vi "Single Shot Camera Test.vi"() -> ()   [LabVIEW 2017]
uses:
  IMAQCV/IMAQCV.lvlib
  IMAQCV/LVOpenCV.lvlib
panel:
  in  "Image Size":T1(ring)
  out "Gray picture":picture
  out "Color picture":picture
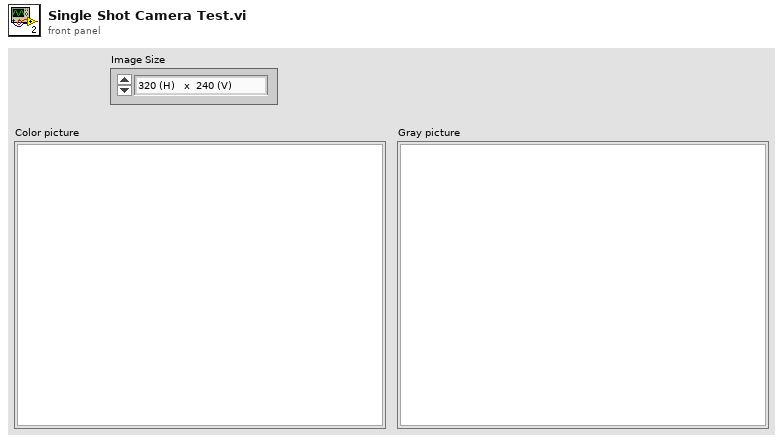
[diagram p1: front panel]
types:
  T1 = enum16{"320 (H)   x  240 (V)", "352(H)    x  288 (V)", "640 (H)   x  480 (V) ", "800 (H)   x  600 (V)", "1024 (H) x  768 (V)", "1280 (H) x  720 (V)", "1280 (H) x  960 (V)", "1280 (H) x 1024 (V)", "1920 (H) x 1080 (V)"}
  T2 = typedef "IMAQCV.lvlib/IMAQCV Image.ctl" = refnum<vi>
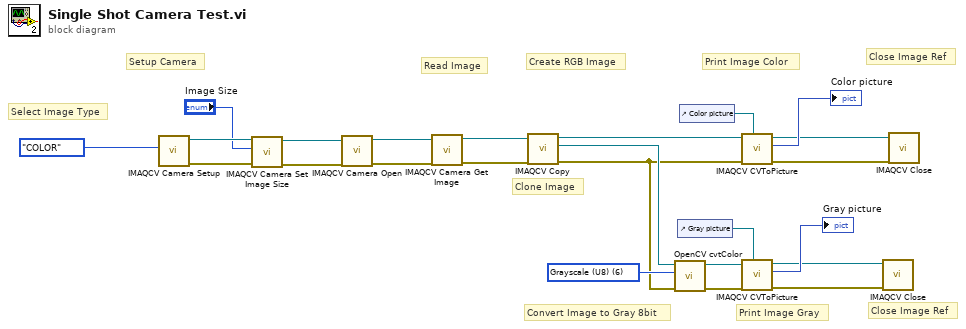
[diagram p0: block diagram]
diagram:
  w17 = u32 6 items=["RGB (U32)"=0, "Grayscale (U8)"=6, "RGB-Grayscale (U8)"=10, "Gray-RGB (U32)"=9] ("code")
  # "Select Image Type"
  # "Print Image Color"
  # "Close Image Ref"
  # "Close Image Ref"
  # "Print Image Gray"
  # "Convert Image to Gray 8bit"
  # "Clone Image"
  # "Create RGB Image"
  # "Read Image"
  # "Setup Camera"
  n1 = call "IMAQCV Camera Setup.vi"("type"=enum16{"GRAY", "COLOR"}."COLOR") -> ("error out"=w24:errorcluster, "image out"=w23:T2)  [unwired: 9 in]
  n2 = call "IMAQCV Camera Set Image Size.vi"("error in (no error)"=w24, "Image Size"="Image Size", "image in"=w23) -> ("error out"=w6:errorcluster, "image out"=w5:T2)  [unwired: 7 in]
  n3 = call "IMAQCV Camera Open.vi"("error in (no error)"=w6, "image in"=w5) -> ("error out"=w22:errorcluster, "image out"=w21:T2)  [unwired: 8 in]
  n4 = call "IMAQCV Camera Get Image.vi"("error in (no error)"=w22, "image in"=w21) -> ("error out"=w19:errorcluster, "image out"=w20:T2)  [unwired: 8 in]
  n5 = call "IMAQCV Copy.vi"("error in (no error)"=w19, "Image Src"=w20) -> ("error out"=w11:errorcluster, "Image Dst Out"=w16:T2, "Image Src Out"=w15:T2)  [unwired: 6 in]
  n6 = call "OpenCV cvtColor.vi"("error in (no error)"=w11, "code"=w17, "image in"=w16) -> ("error out"=w14:errorcluster, "image out"=w13:T2)  [unwired: 7 in]
  n7 = control-ref of="Gray picture"() -> (w3:refnum<vi>)
  n8 = control-ref of="Color picture"() -> (w4:refnum<vi>)
  n9 = call "IMAQCV CVToPicture.vi"("picture ref"=w4, "error in (no error)"=w11, "image"=w15) -> ("error out"=w10:errorcluster, "picture"=→"Color picture":picture, "image out"=w9:T2)  [unwired: 6 in]
  n10 = call "IMAQCV CVToPicture.vi"("picture ref"=w3, "error in (no error)"=w14, "image"=w13) -> ("error out"=w8:errorcluster, "picture"=→"Gray picture":picture, "image out"=w7:T2)  [unwired: 6 in]
  n11 = call "IMAQCV Close.vi"("error in (no error)"=w8, "Image"=w7) -> ()  [unwired: 9 in, 1 out]
  n12 = call "IMAQCV Close.vi"("error in (no error)"=w10, "Image"=w9) -> ()  [unwired: 9 in, 1 out]
